vi "Close Font.vi"(8 "error in (no error)":errorcluster, 11 "Font Pointer":u32 format="%.0x") -> (0 "error out":errorcluster)   [LabVIEW 2015, in "LibSDL2_TTF.lvlib"]
uses:
  LibSDL2_TTF.lvlib
  LibSDL2 Wrapper/DLL/SDL2_ttf.dll
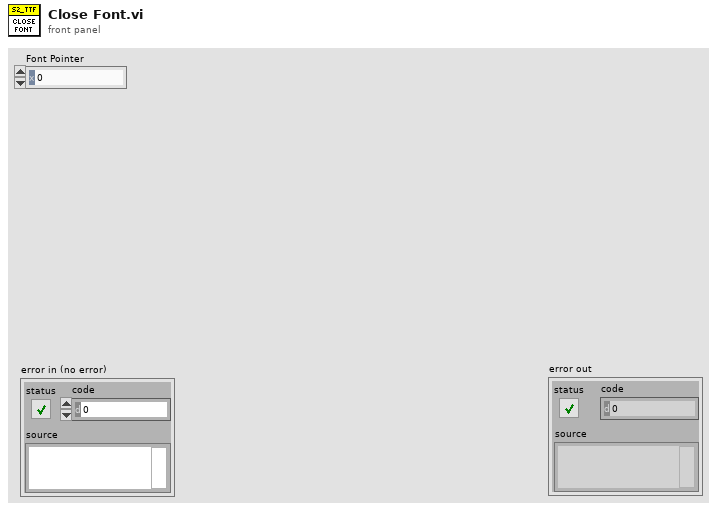
[diagram p1: front panel]
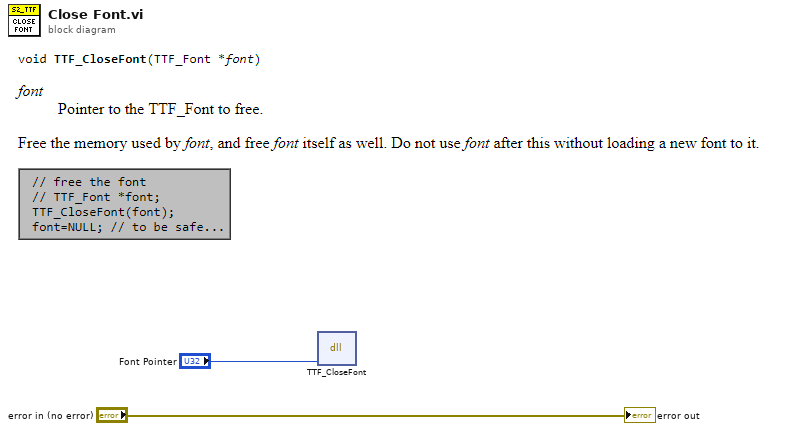
[diagram p0: block diagram]
diagram:
  n1 = dll-call lib="C:/dev/PGS/LabSDL2/Source/Libraries/LibSDL2 Wrapper/DLL/SDL2_ttf.dll" fn="TTF_CloseFont"("Font"="Font Pointer") -> ()  [unwired: 5 in, 2 out]
  "error out" <- "error in (no error)"
